vi "working_interface.vi"(10 "VISA resource name":refnum<visa-resource-name>="TRIG") -> (2 "data in delay generator (s)":dbl[](array[numeric]) caption="delay array" min=0.0 max=2000.0 format="%.3f")   [LabVIEW 2011]
panel:
  in  "time unit":enum16{"s", "ms", "us", "ns"}(ring)=enum."us"
  in  "resolution":i32=100
  in  "duration array":dbl[](array[numeric]) format="%.3f"
  in  "start time array":dbl[](array[numeric]) format="%.3f"
  out "Digital Waveform Graph":digitalwaveform(graph)
  in  "trigger":bool
  in  "write data":bool
  in  "read delay data":bool
  in  "stop":bool
  # "timing values are only relative,\n the absolute values are given in the\ndelay array!!!\n\nt0 and t can not be written to the device, t0 is always 0\nand  t is always the longest time + 25ns. However, t is \nused to display how long the nozzle is open to give a real \nrepresentation in the diagram (and only there). \nYou can change that time to pretty much any value, \nbut the nozzle itself is not controlled through the labview\n software. You have to set the time manually at the \nnozzle driver and ideally you should then enter that time\nfor t as well!\n\ndelay array index:\n0 - t0 = nozzle start (TTL) = 0\n1 - nozzle duration\n2 - power AMP START\n3 - power AMP STOP\n4 - AWG START (TTL)\n5 - AWG STOP (NA)\n6 - SWITCH ON \n7 - SWITCH OFF\n8 - OSC START (TTL)\n9 - OSC STOP (NA)\n\nTTL -> tool starts on rising flank\nof signal, hence the falling flank \nand the duration are not important!"
  # "delay array index:\n0 - to = nozzle start (TTL) = 0\n1 - t = nozzle duration\n2 - A = power AMP START\n3 - B = power AMP STOP\n4 - C = AWG START (TTL)\n5 - D = AWG STOP (NA)\n6 - E = SWITCH ON \n7 - F = SWITCH OFF\n8 - G = OSC START (TTL)\n9 - H = OSC STOP (NA)\n\nTTL -> tool starts on rising flank\nof signal, hence the falling flank \nand the duration are not important!"
  # "the graph does not show the actual TTL signal for all signals. For those with negative polarity it shows the inverse of the signal \nit shows when everything is active"
  # "t0 is always 0"
  # "AWG must start after power AMP is on \nand while it is still on!"
  # "SWITCH must NOT switch ON before \npower AMP is off!"
  # "t0"
  # "t"
  # "A"
  # "B"
  # "C"
  # "D"
  # "E"
  # "F"
  # "G"
  # "H"
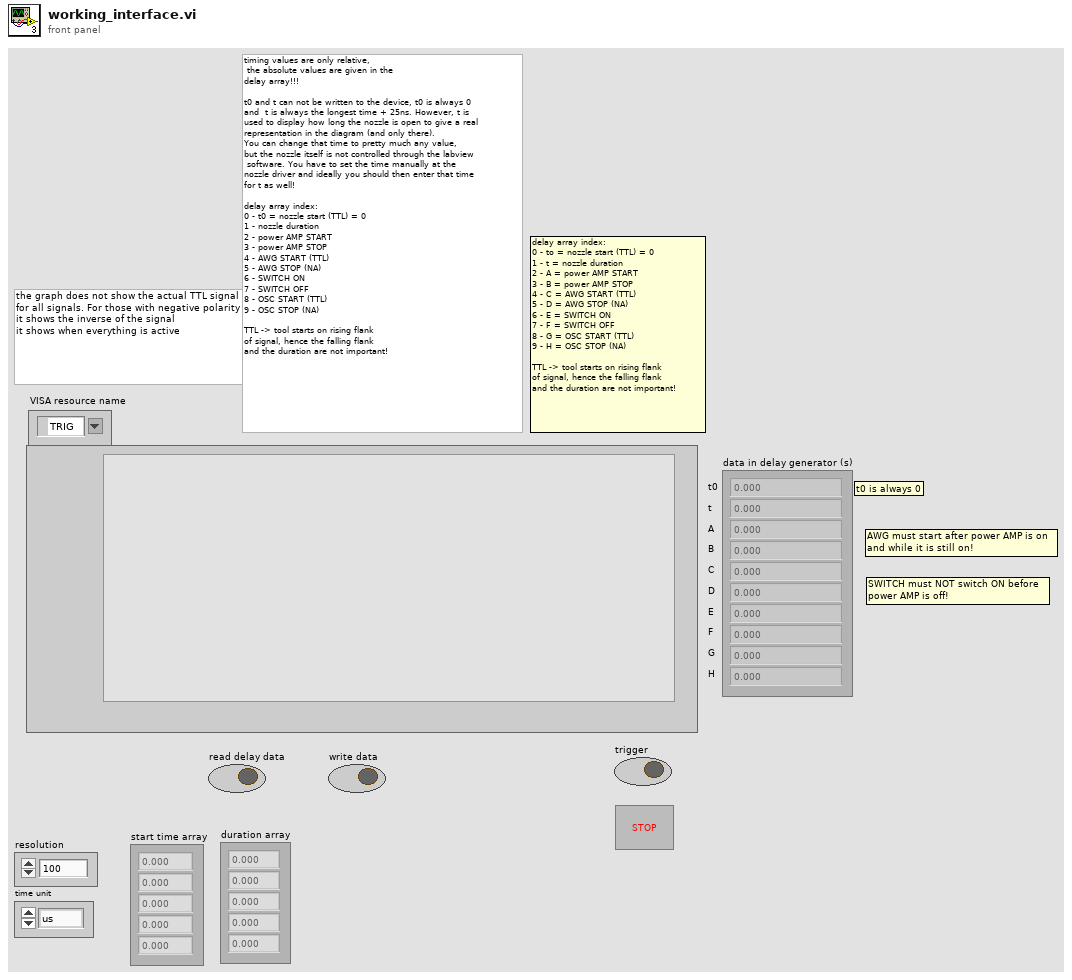
[diagram p1: front panel]
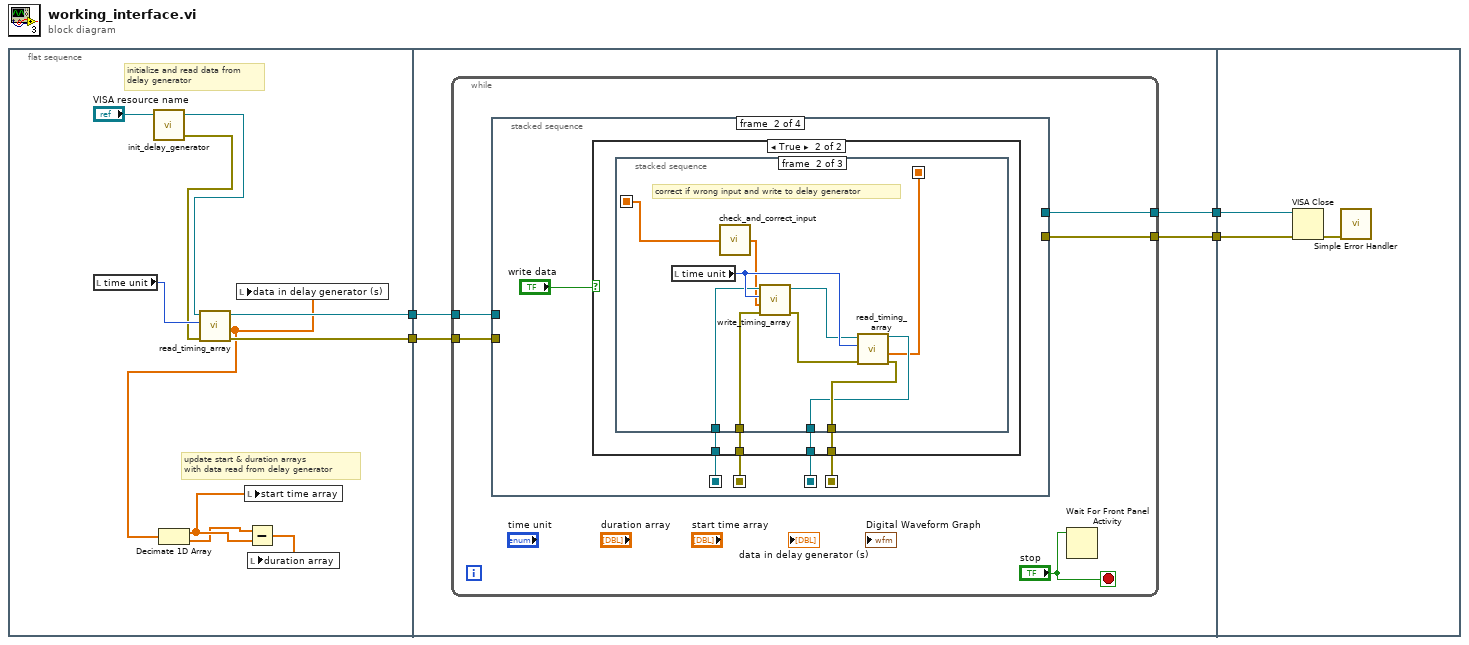
[diagram p0: block diagram]
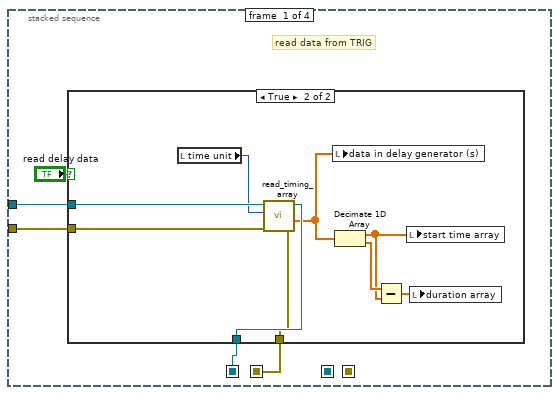
[diagram p2: hidden frame]
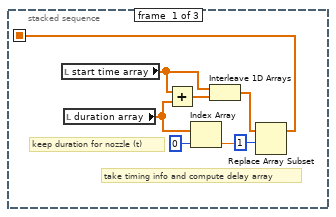
[diagram p5: hidden frame]
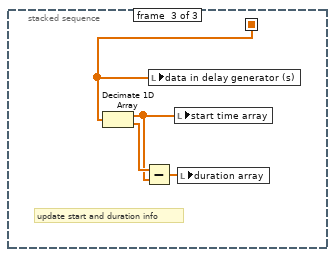
[diagram p6: hidden frame]
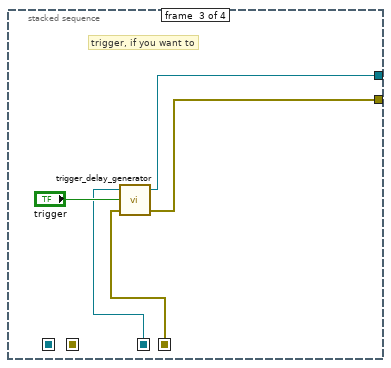
[diagram p7: hidden frame]
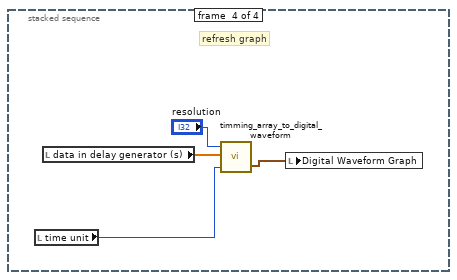
[diagram p8: hidden frame]
diagram:
  n1 = flat-sequence {
    tunnel: [w13] -> w4
    tunnel: [w14] -> w3
    tunnel: w4 -> [w18]
    tunnel: w3 -> [w17]
    tunnel: [w16] -> w2
    tunnel: [w15] -> w1
    tunnel: w2 -> [w84]
    tunnel: w1 -> [w83]
    frame #0 {
      # "update start & duration arrays \nwith data read from delay generator"
      # "initialize and read data from \ndelay generator"
      n2 = local read "time unit"() -> (w9:enum16{"s", "ms", "us", "ns"})
      n3 = call "init_delay_generator.vi"("VISA resource name"="VISA resource name") -> ("error out"=w5:errorcluster, "VISA resource name out"=w6:refnum<visa-resource-name>)  [unwired: 3 in]
      n4 = call "read_timing_array.vi"("error in"=w5, "time unit"=w9, "VISA resource in"=w6) -> ("error out 2"=w14:errorcluster, "delay array"=w8:dbl[], "VISA resource out"=w13:refnum<visa-resource-name>)  [unwired: 2 in]
      n5 = Decimate 1D Array(w8) -> (w11:dbl[], w10:dbl[])
      n6 = local write "data in delay generator (s)"(w8) -> ()
      n7 = local write "start time array"(w11) -> ()
      n8 = Subtract(x=w10, y=w11) -> (x-y=w12:dbl[])
      n9 = local write "duration array"(w12) -> ()
    }
    frame #1 {
      n10 = while {
        tunnel: w17 -> [w21]
        tunnel: [w23] -> w16
        tunnel: [w22] -> w15
        tunnel: w18 -> [w19]
        stop <- "stop" stop-if-true
        n11 = stacked-sequence {
          seq-local: [w26 _ _ _] -> [_ w41 _ _]
          seq-local: [w25 _ _ _] -> [_ w40 _ _]
          seq-local: [_ w43 _ _] -> [_ _ w74 _]
          seq-local: [_ w42 _ _] -> [_ _ w75 _]
          tunnel: w19 -> [w28 _ _ _]
          tunnel: w21 -> [w27 _ _ _]
          tunnel: [_ _ w73 _] -> w22
          tunnel: [_ _ w77 _] -> w23
          frame #0 {
            # "read data from TRIG"
            n12 = case shown="True" "read delay data" {
              tunnel: w28 -> [w29 w39]
              tunnel: w27 -> [w30 w38]
              tunnel: [w29 w37] -> w26
              tunnel: [w30 w36] -> w25
              frame False {
              }
              frame True {
                n13 = local read "time unit"() -> (w35:enum16{"s", "ms", "us", "ns"})
                n14 = call "read_timing_array.vi"("error in"=w38, "time unit"=w35, "VISA resource in"=w39) -> ("error out 2"=w36:errorcluster, "delay array"=w32:dbl[], "VISA resource out"=w37:refnum<visa-resource-name>)  [unwired: 2 in]
                n15 = local write "data in delay generator (s)"(w32) -> ()
                n16 = Decimate 1D Array(w32) -> (w31:dbl[], w33:dbl[])
                n17 = Subtract(x=w33, y=w31) -> (x-y=w34:dbl[])
                n18 = local write "start time array"(w31) -> ()
                n19 = local write "duration array"(w34) -> ()
              }
            }
          }
          frame #1 {
            n20 = case shown="True" "write data" {
              tunnel: [w46 w47] -> w43
              tunnel: [w45 w50] -> w42
              tunnel: w41 -> [w46 w49]
              tunnel: w40 -> [w45 w48]
              frame False {
              }
              frame True {
                n21 = stacked-sequence {
                  seq-local: [w51 _ _] -> [_ w61 _]
                  seq-local: [_ w60 _] -> [_ _ w70]
                  tunnel: [_ w68 _] -> w50
                  tunnel: w49 -> [_ w66 _]
                  tunnel: w48 -> [_ w65 _]
                  tunnel: [_ w62 _] -> w47
                  frame #0 {
                    # "take timing info and compute delay array"
                    # "keep duration for nozzle (t)"
                    n22 = local read "start time array"() -> (w57:dbl[])
                    n23 = local read "duration array"() -> (w56:dbl[])
                    n24 = Add(x=w57, y=w56) -> (x+y=w58:dbl[])
                    n25 = Index Array(array=w56, index=0) -> (element=w52:dbl)
                    n26 = Interleave 1D Arrays(w57, w58) -> (w54:dbl[])
                    n27 = Replace Array Subset(array=w54, new element=w52, index=1) -> (w51:dbl[])
                  }
                  frame #1 {
                    # "correct if wrong input and write to delay generator"
                    n28 = local read "time unit"() -> (w67:enum16{"s", "ms", "us", "ns"})
                    n29 = call "check_and_correct_input.vi"("delay array"=w61) -> ("corrrected delay array"=w59:dbl[])  [unwired: 4 in]
                    n30 = call "write_timing_array.vi"("error in"=w65, "delay array"=w59, "time unit"=w67, "VISA resource in"=w66) -> ("error out 2"=w63:errorcluster, "VISA resource out"=w64:refnum<visa-resource-name>)  [unwired: 2 in]
                    n31 = call "read_timing_array.vi"("error in"=w63, "time unit"=w67, "VISA resource in"=w64) -> ("error out 2"=w68:errorcluster, "delay array"=w60:dbl[], "VISA resource out"=w62:refnum<visa-resource-name>)  [unwired: 2 in]
                  }
                  frame #2 {
                    # "update start and duration info"
                    n32 = Decimate 1D Array(w70) -> (w69:dbl[], w72:dbl[])
                    n33 = Subtract(x=w72, y=w69) -> (x-y=w71:dbl[])
                    n34 = local write "data in delay generator (s)"(w70) -> ()
                    n35 = local write "start time array"(w69) -> ()
                    n36 = local write "duration array"(w71) -> ()
                  }
                }
              }
            }
          }
          frame #2 {
            # "trigger, if you want to"
            n37 = call "trigger_delay_generator.vi"("error in (no error)"=w75, "Boolean"="trigger", "VISA resource name"=w74) -> ("error out"=w73:errorcluster, "VISA resource name 2"=w77:refnum<visa-resource-name>)  [unwired: 1 in]
          }
          frame #3 {
            # "refresh graph"
            n38 = local read "time unit"() -> (w78:enum16{"s", "ms", "us", "ns"})
            n39 = local read "data in delay generator (s)"() -> (w81:dbl[])
            n40 = call "timming_array_to_digital_waveform.vi"("time unit"=w78, "delay array"=w81, "resolution"="resolution") -> ("digital waveform"=w80:digitalwaveform)  [unwired: 1 in]
            n41 = local write "Digital Waveform Graph"(w80) -> ()
          }
        }
        n42 = Wait For Front Panel Activity(3:"stop") -> ()  [unwired: 2 in, 1 out]
      }
    }
    frame #2 {
      n43 = VISA Close(VISA resource name=w84, error in (no error)=w83) -> (error out=w82:errorcluster)
      n44 = call <vilib>:"Simple Error Handler.vi"("error in (no error)"=w82) -> ()  [unwired: 4 in, 5 out]
    }
  }
